vi "TempMonitor_TempToVoltage.vi"(2 "Max Voltage":dbl=5.0, 3 "Min Voltage":dbl, 5 "Temp (C)":dbl) -> (0 "Temp Outside Voltage Limits":bool, 1 "Output Voltage":dbl)   [LabVIEW 2012]
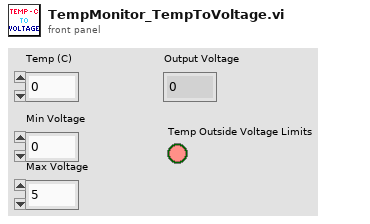
[diagram p1: front panel]
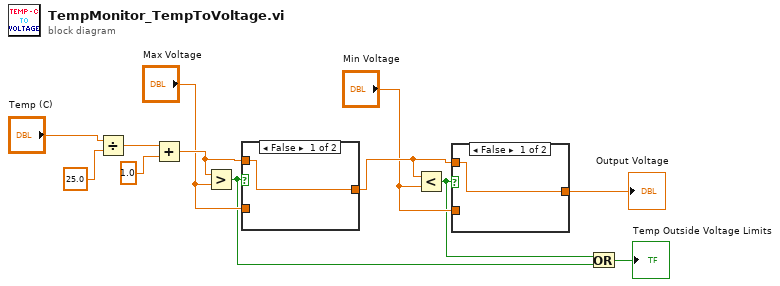
[diagram p0: block diagram]
diagram:
  n1 = Divide(x="Temp (C)", y=25.0) -> (x/y=w10:dbl)
  n2 = Add(x=w10, y=1.0) -> (x+y=w8:dbl)
  n3 = Greater?(x=w8, y="Max Voltage") -> (0:w1:bool)
  n4 = case shown="False" w1 {
    tunnel: w8 -> [w13 _]
    tunnel: "Max Voltage" -> [_ w14]
    tunnel: [w13 w14] -> w6
    frame False {
    }
    frame True {
    }
  }
  n5 = Less?(x=w6, y="Min Voltage") -> (x < y?=w2:bool)
  n6 = case shown="False" w2 {
    tunnel: w6 -> [w15 _]
    tunnel: "Min Voltage" -> [_ w16]
    tunnel: [w15 w16] -> w4
    frame False {
    }
    frame True {
    }
  }
  "Output Voltage" <- w4
  n7 = Or(x=w2, y=w1) -> (x .or. y?=→"Temp Outside Voltage Limits":bool)
